vi "CLD 11 Producer consumer events front panel.vi"() -> ()   [LabVIEW 2025]
doc: "CLD 11 exercise"
uses:
  CLD 11 Producer Consumer Data Structure.ctl
  CLD 11 CSV file data structure.ctl
  CLD 11 producer consumer enum.ctl
  CLD 11 CSV file enum.ctl
panel:
  out "Current Time target":dbl
  out "Step 3":bool
  out "Step 2":bool
  out "Step 1":bool
  out "Time Has Elapsed":bool
  out "Elapsed Time":string
  in  "Auto Reset":bool=TRUE
  in  "Reset Button":bool
  in  "Stop VI":bool
  in  "Time Target (s)":dbl
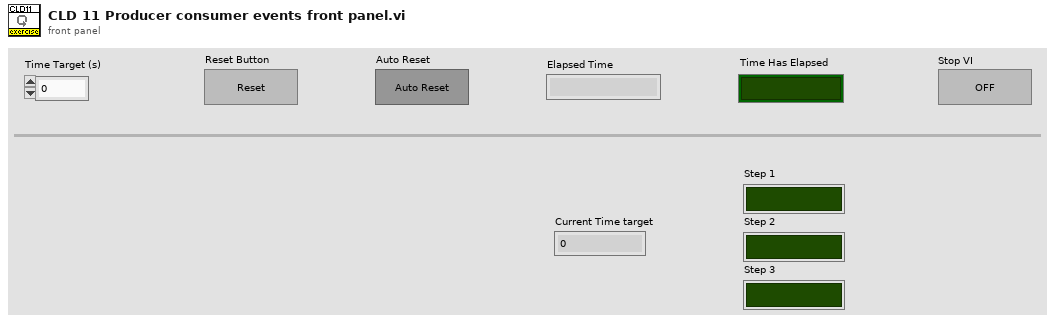
[diagram p1: front panel]
types:
  T1 = typedef "CLD 11 producer consumer enum.ctl" = enum16{"Initialize App", "Read CSV File", "Check Timer", "Run State One", "Run State Two", "Run State Three", "Stop App", "Reset", "Autoreset"}
  T2 = typedef "CLD 11 Producer Consumer Data Structure.ctl" = cluster{"CSV File Data Structure":T3, "Time has Elapsed":bool, "Reset":bool, "Autoreset":bool, "Time Target (s)":dbl, "Current State Number":i32}
  T3 = typedef "CLD 11 CSV file data structure.ctl" = cluster{"Dwell Time":i32, "State 1":bool, "State 2":bool, "State 3":bool}
  T4 = typedef "CLD 11 CSV file enum.ctl" = enum16{"Read CSV", "Write CSV"}
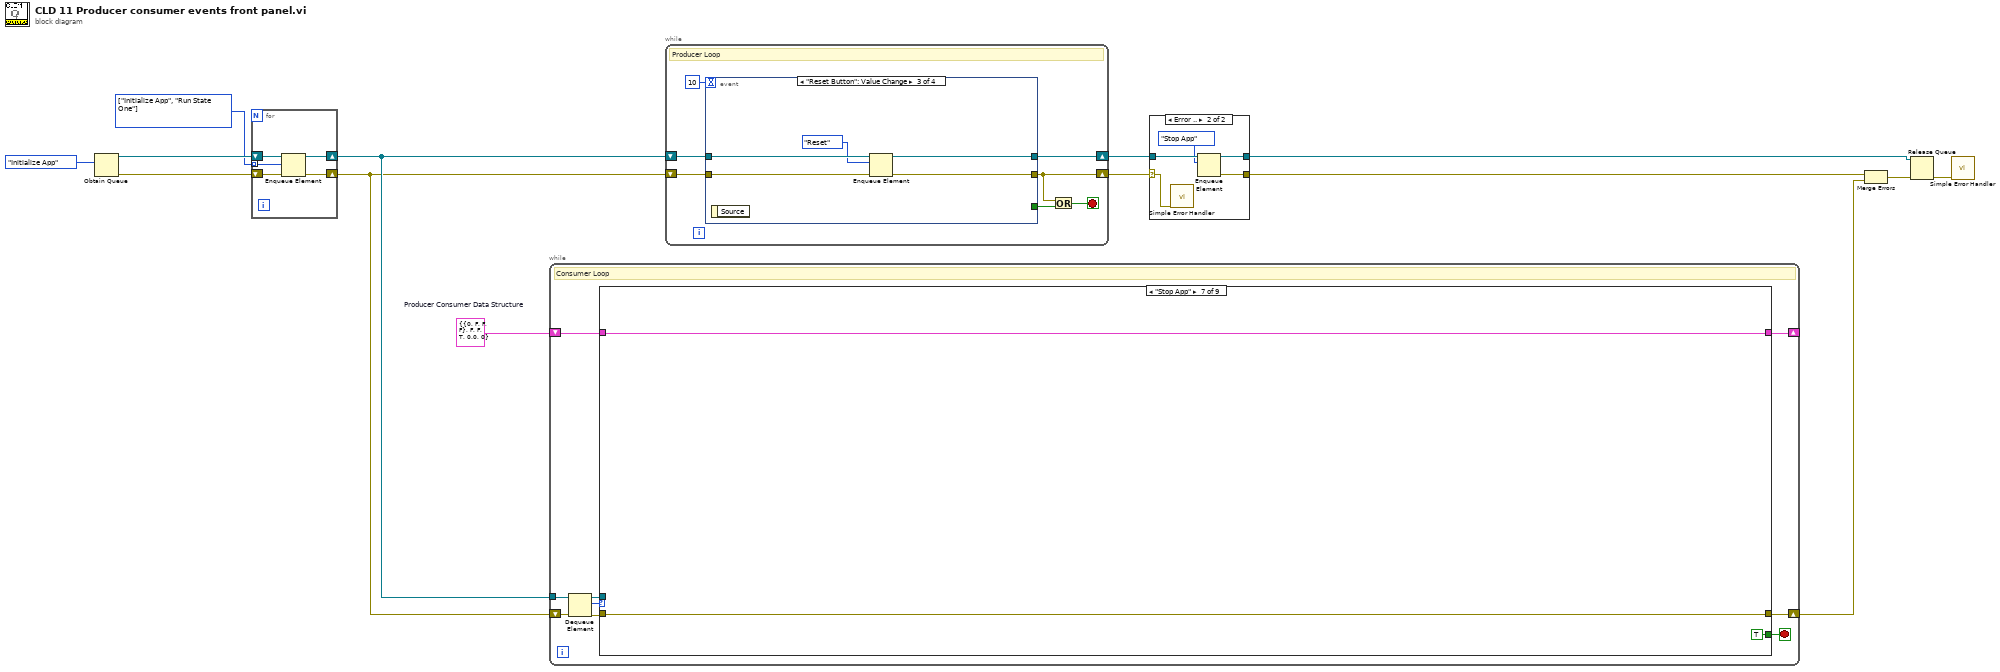
[diagram p0: block diagram]
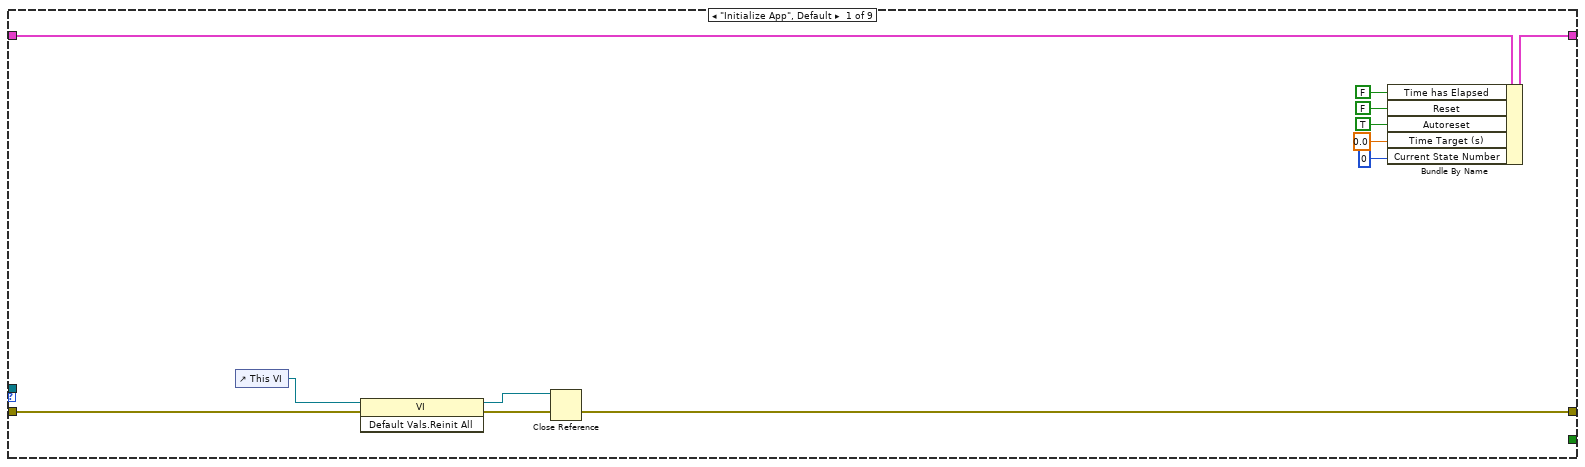
[diagram p3: hidden frame]
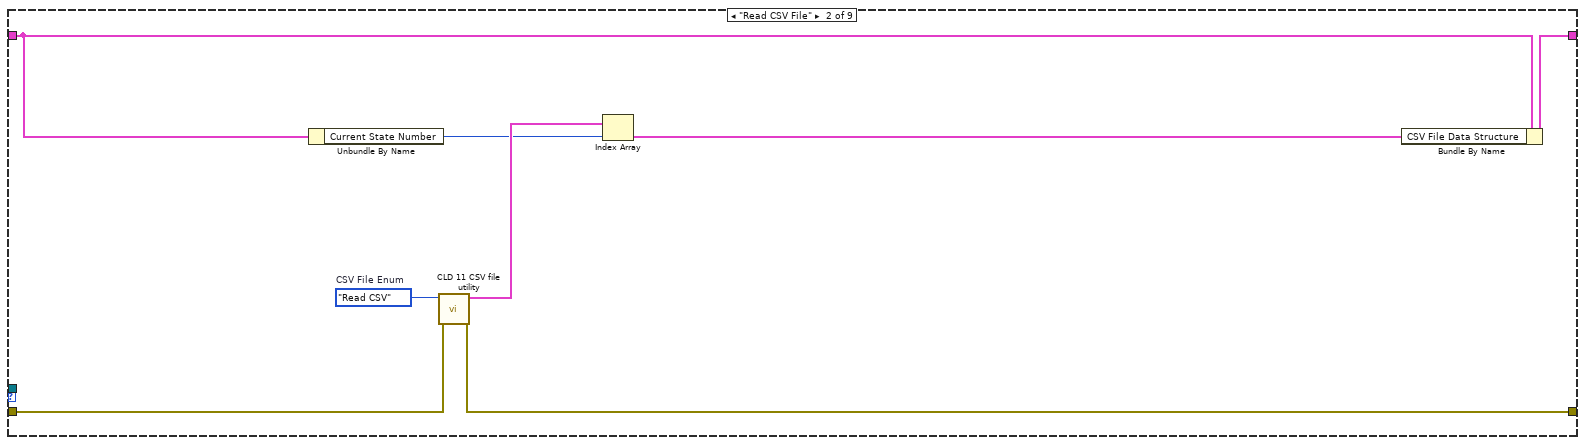
[diagram p4: hidden frame]
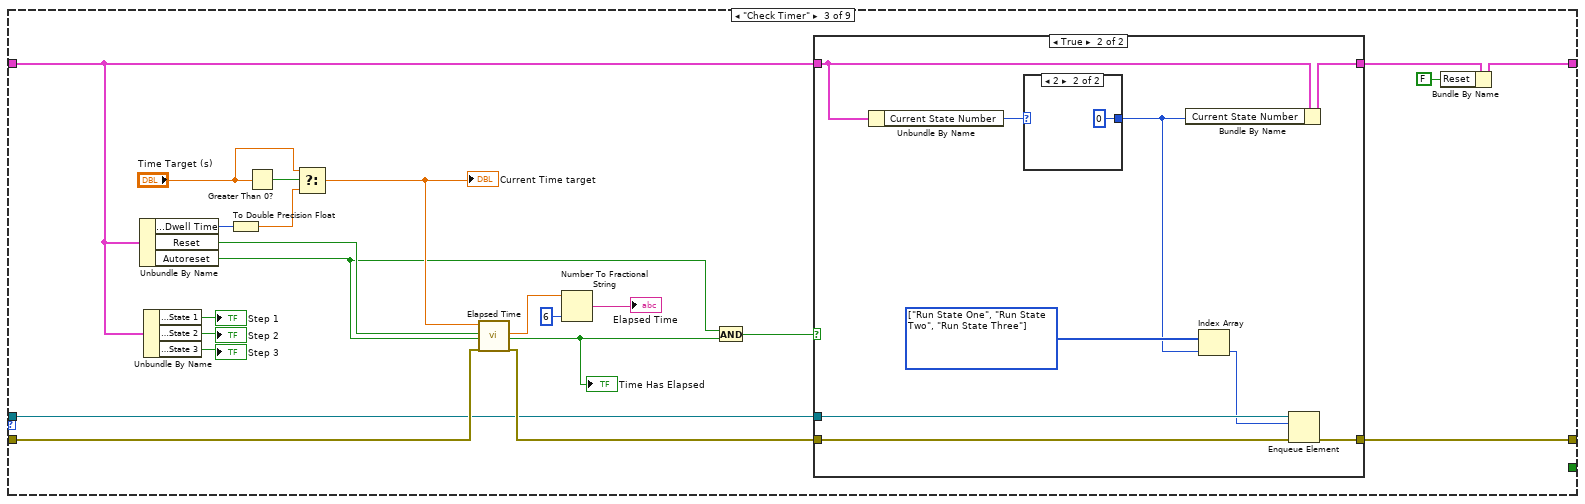
[diagram p5: hidden frame]
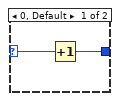
[diagram p7: hidden frame]
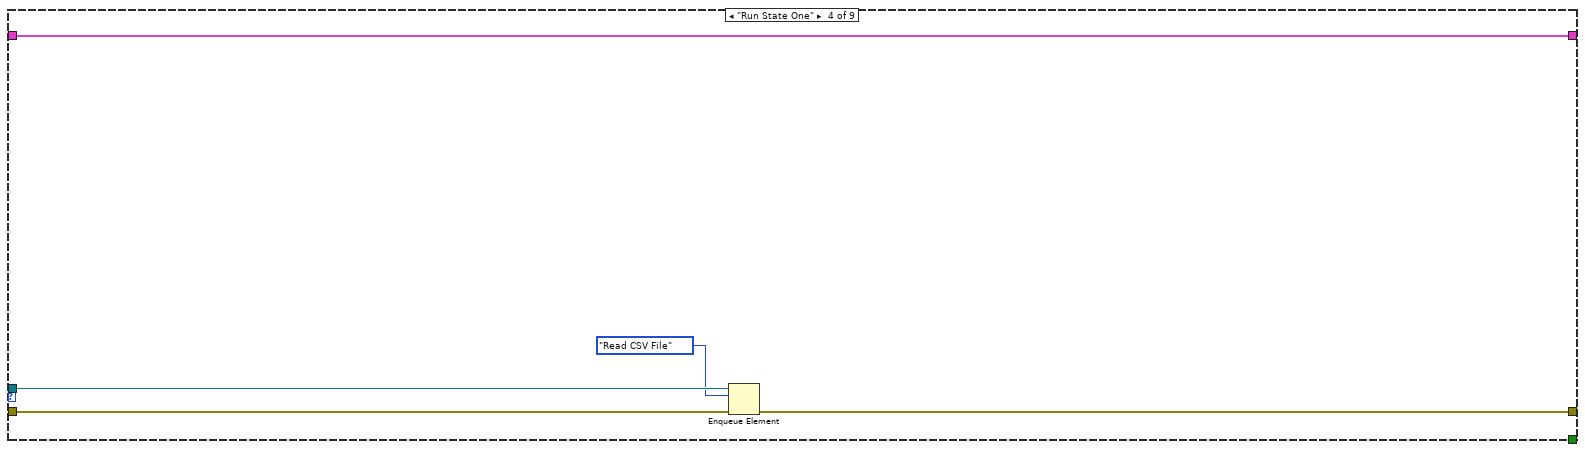
[diagram p8: hidden frame]
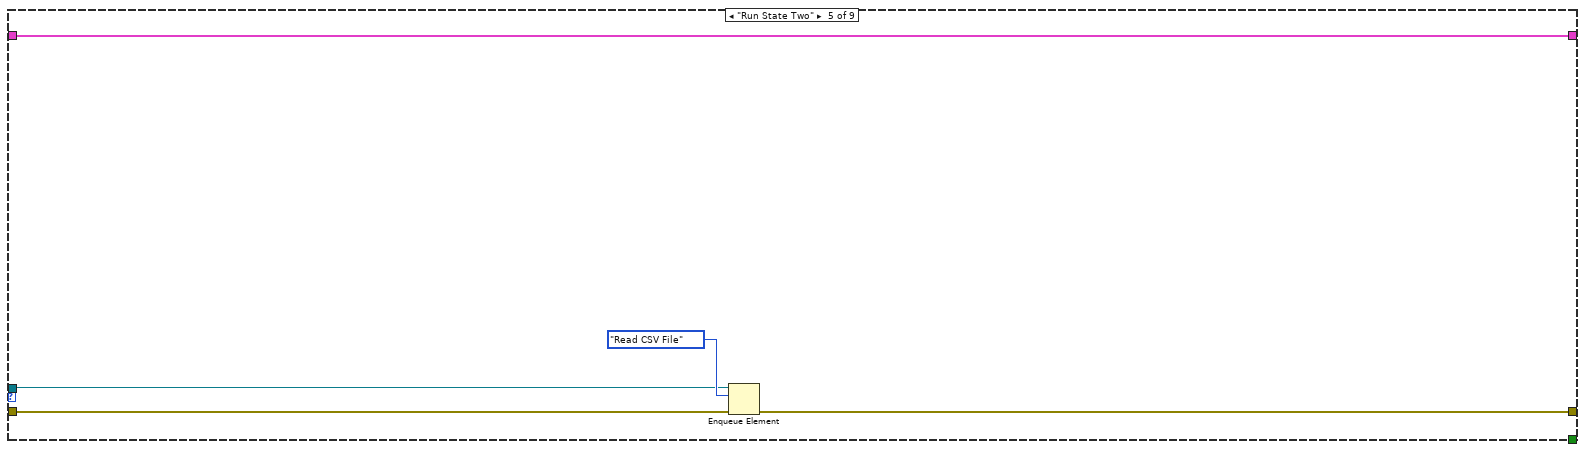
[diagram p9: hidden frame]
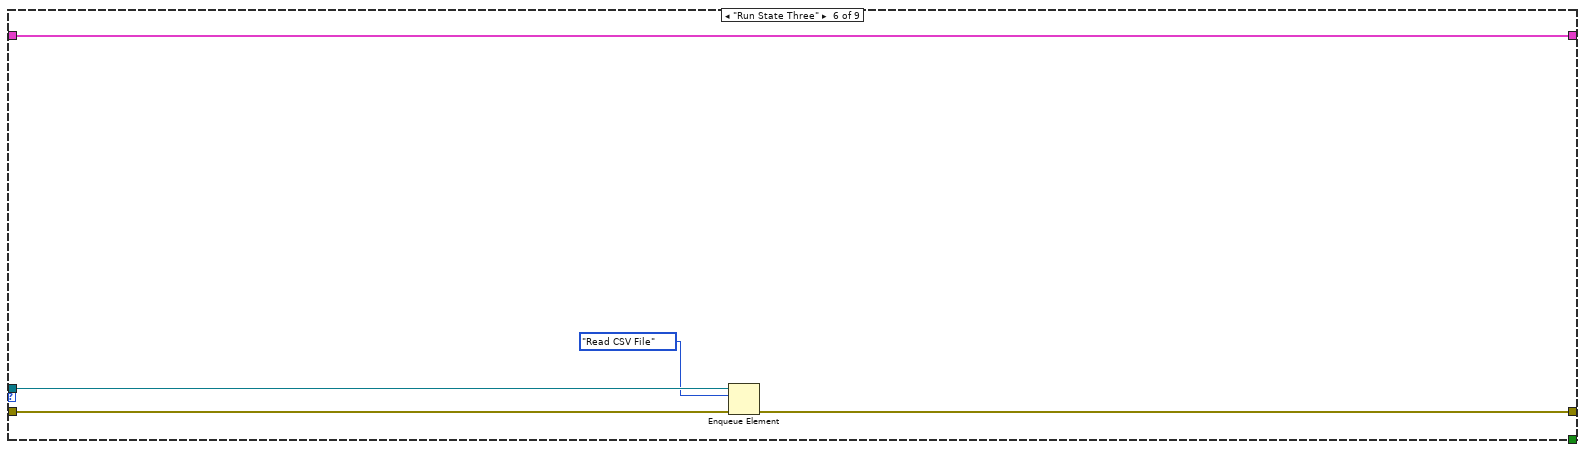
[diagram p10: hidden frame]
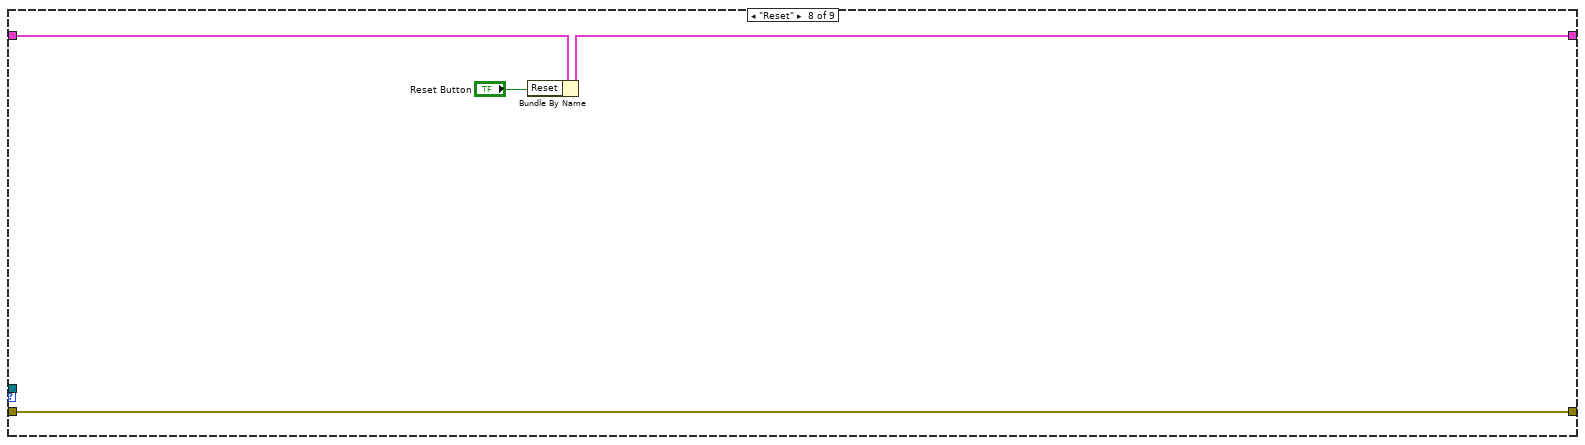
[diagram p11: hidden frame]
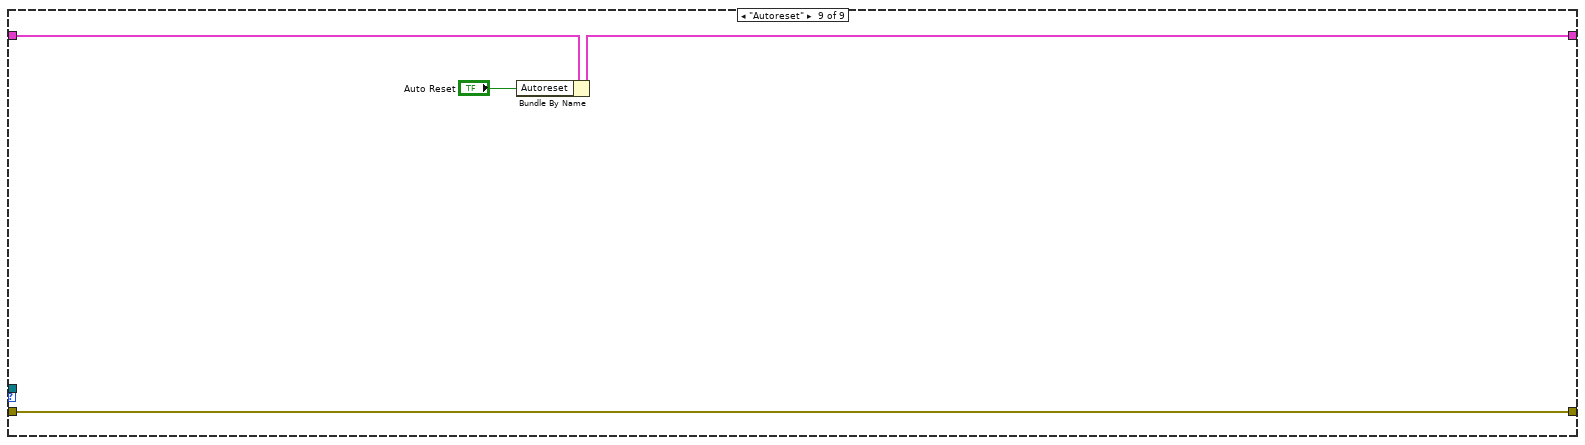
[diagram p12: hidden frame]
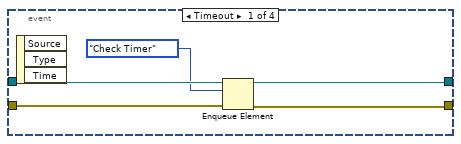
[diagram p13: hidden frame]
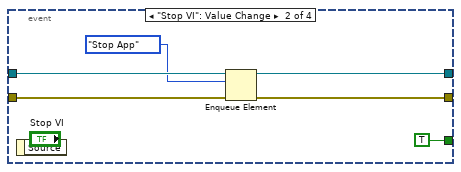
[diagram p14: hidden frame]
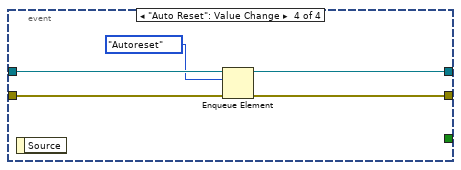
[diagram p15: hidden frame]
diagram:
  w8 = T1[] [enum."Initialize App", enum."Run State One"] items=["Initialize App", "Read CSV File", "Check Timer", "Run State One", "Run State Two", "Run State Three", "Stop App", "Reset", "Autoreset"] ("element")
  w14 = T2 {"CSV File Data Structure"={"Dwell Time"=0, "State 1"=FALSE, "State 2"=FALSE, "State 3"=FALSE}, "Time has Elapsed"=FALSE, "Reset"=FALSE, "Autoreset"=TRUE, "Time Target (s)"=0.0, "Current State Number"=0}  # Producer Consumer Data Structure
  n1 = Obtain Queue(element data type=CLD_11_producer_consumer_enum."Initialize App" ("CLD 11 Timer Enum")) -> (queue out=w11:refnum<queue>, error out=w12:errorcluster)  [unwired: 4 in, 1 out]
  n2 = for {
    shift-right: [w18] -> w9
    shift-left: w12 -> [w19]
    shift-right: [w16] -> w10
    shift-left: w11 -> [w17]
    tunnel: w8 -> [w15] mode=indexing
    n3 = Enqueue Element(queue=w17, element=w15, error in (no error)=w19) -> (queue out=w16:refnum<queue>, error out=w18:errorcluster)  [unwired: 1 in, 1 out]
  }
  n4 = while {
    shift-right: [w26] -> _
    shift-left: w14 -> [w28]
    tunnel: w10 -> [w27]
    shift-right: [w21] -> w7
    shift-left: w9 -> [w23]
    stop <- w24 stop-if-true
    # "Consumer Loop"
    n5 = Dequeue Element(queue=w27, error in (no error)=w23) -> (queue out=w20:refnum<queue>, element=w25:T1, error out=w22:errorcluster)  [unwired: 1 in, 1 out]
    n6 = case shown="\"Stop App\"" w25 {
      tunnel: w28 -> [w40 w44 w55 w90 w95 w97 w103 w107 w111]
      tunnel: [w34 w45 w50 w90 w95 w97 w103 w105 w109] -> w26
      tunnel: [_ _ _ _ _ _ TRUE _ _] -> w24
      tunnel: w22 -> [w39 w48 w71 w89 w94 w100 w101 w106 w110]
      tunnel: [w36 w47 w52 w88 w93 w99 w101 w106 w110] -> w21
      tunnel: w20 -> [_ _ w51 w87 w91 w98 _ _ _]
      frame "Initialize App", Default {
        n7 = control-ref of="This VI"() -> (w37:refnum<vi>)
        n8 = invoke class="VI" method="Default Vals.Reinit All"(reference=w37, error in=w39) -> (reference out=w35:refnum<vi>, error out=w38:errorcluster)  [unwired: 1 in, 1 out]
        n9 = Close Reference(reference=w35, error in (no error)=w38) -> (error out=w36:errorcluster)
        n10 = Bundle By Name(cluster=w40, "Time has Elapsed"=FALSE, "Reset"=FALSE, "Autoreset"=TRUE, "Time Target (s)"=0.0, "Current State Number"=0) -> (w34:T2)
      }
      frame "Read CSV File" {
        w46 = CLD_11_CSV_file_enum."Read CSV"  # CSV File Enum
        n11 = Unbundle By Name(w44) -> ("Current State Number"=w42:i32)
        n12 = call "CLD 11 CSV file utility.vi"("Error In"=w48, "CSV File Enum"=w46) -> ("Error Out"=w47:errorcluster, "[Data Out]"=w43:T3[])  [unwired: 8 in]
        n13 = Index Array(array=w43, index=w42) -> (element=w41:T3)
        n14 = Bundle By Name(cluster=w44, "CSV File Data Structure"=w41) -> (w45:T2)
      }
      frame "Check Timer" {
        n15 = Unbundle By Name(w55) -> ("CSV File Data Structure.Dwell Time"=w61:i32, "Reset"=w64:bool, "Autoreset"=w57:bool)
        n16 = Unbundle By Name(w55) -> ("CSV File Data Structure.State 1"=→"Step 1":bool, "CSV File Data Structure.State 2"=→"Step 2":bool, "CSV File Data Structure.State 3"=→"Step 3":bool)
        n17 = To Double Precision Float(number=w61) -> (double precision float=w60:dbl)
        n18 = Greater Than 0?(x="Time Target (s)") -> (x > 0?=w63:bool)
        n19 = Select(t="Time Target (s)", s=w63, f=w60) -> (s? t:f=w59:dbl)
        "Current Time target" <- w59
        n20 = call "Elapsed Time"("Time Target (s)"=w59, "Reset"=w64, "Auto Reset"=w57, "error in (no error)"=w71) -> ("Elapsed Time (s)"=w66:dbl, "Time has Elapsed"=w58:bool, "error out"=w53:errorcluster)  [unwired: 8 in, 5 out]
        "Time Has Elapsed" <- w58
        n21 = Number To Fractional String(number=w66, precision (6)=i16 6) -> (F-format string=→"Elapsed Time":string)  [unwired: 2 in]
        n22 = And(x=w57, y=w58) -> (x .and. y?=w56:bool)
        n23 = case shown="True" w56 {
          tunnel: w55 -> [w73 w81]
          tunnel: [w73 w82] -> w54
          tunnel: w53 -> [w72 w79]
          tunnel: [w72 w78] -> w52
          tunnel: w51 -> [_ w77]
          frame False {
          }
          frame True {
            w76 = T1[] [enum."Run State One", enum."Run State Two", enum."Run State Three"] items=["Initialize App", "Read CSV File", "Check Timer", "Run State One", "Run State Two", "Run State Three", "Stop App", "Reset", "Autoreset"] ("element")
            n24 = Unbundle By Name(w81) -> ("Current State Number"=w80:i32)
            n25 = case shown="2" w80 {
              selector: w80 -> [w84 _]
              tunnel: [w83 0] -> w75
              frame 0, Default {
                n26 = Increment(x=w84) -> (x+1=w83:i32)
              }
              frame 2 {
              }
            }
            n27 = Bundle By Name(cluster=w81, "Current State Number"=w75) -> (w82:T2)
            n28 = Index Array(array=w76, index=w75) -> (element=w74:T1)
            n29 = Enqueue Element(queue=w77, element=w74, error in (no error)=w79) -> (error out=w78:errorcluster)  [unwired: 1 in, 2 out]
          }
        }
        n30 = Bundle By Name(cluster=w54, "Reset"=FALSE) -> (w50:T2)
      }
      frame "Run State One" {
        n31 = Enqueue Element(queue=w87, element=CLD_11_producer_consumer_enum."Read CSV File", error in (no error)=w89) -> (error out=w88:errorcluster)  [unwired: 1 in, 2 out]
      }
      frame "Run State Two" {
        n32 = Enqueue Element(queue=w91, element=CLD_11_producer_consumer_enum."Read CSV File", error in (no error)=w94) -> (error out=w93:errorcluster)  [unwired: 1 in, 2 out]
      }
      frame "Run State Three" {
        n33 = Enqueue Element(queue=w98, element=CLD_11_producer_consumer_enum."Read CSV File", error in (no error)=w100) -> (error out=w99:errorcluster)  [unwired: 1 in, 2 out]
      }
      frame "Stop App" {
      }
      frame "Reset" {
        n34 = Bundle By Name(cluster=w107, "Reset"="Reset Button") -> (w105:T2)
      }
      frame "Autoreset" {
        n35 = Bundle By Name(cluster=w111, "Autoreset"="Auto Reset") -> (w109:T2)
      }
    }
  }
  n36 = while {
    shift-right: [w114] -> w3
    shift-left: w10 -> [w118]
    shift-right: [w112] -> w5
    shift-left: w9 -> [w117]
    stop <- w113 stop-if-true
    # "Producer Loop"
    n37 = event shown="[2] \"Reset Button\": Value Change" {
      selector: _ -> [_ _ _ _]
      dyn-events: _ -> [_ _ _ _]
      timeout: 10 -> [_ _ _ _]
      tunnel: w118 -> [w122 w129 w134 w138]
      tunnel: w117 -> [w123 w128 w133 w139]
      tunnel: [_ TRUE _ _] -> w116
      tunnel: [w119 w124 w130 w136] -> w112
      tunnel: [w120 w125 w131 w135] -> w114
      event Timeout {
        n38 = event-data() -> ()  [unwired: 1 in, 3 out]
        n39 = Enqueue Element(queue=w122, element=CLD_11_producer_consumer_enum."Check Timer", error in (no error)=w123) -> (queue out=w120:refnum<queue>, error out=w119:errorcluster)  [unwired: 1 in, 1 out]
      }
      event "Stop VI": Value Change {
        n40 = event-data() -> ()  [unwired: 1 in, 1 out]
        n41 = Enqueue Element(queue=w129, element=CLD_11_producer_consumer_enum."Stop App" ("CLD 11 Timer Enum"), error in (no error)=w128) -> (queue out=w125:refnum<queue>, error out=w124:errorcluster)  [unwired: 1 in, 1 out]
      }
      event "Reset Button": Value Change {
        n42 = event-data() -> ()  [unwired: 1 in, 1 out]
        n43 = Enqueue Element(queue=w134, element=CLD_11_producer_consumer_enum."Reset", error in (no error)=w133) -> (queue out=w131:refnum<queue>, error out=w130:errorcluster)  [unwired: 1 in, 1 out]
      }
      event "Auto Reset": Value Change {
        n44 = event-data() -> ()  [unwired: 1 in, 1 out]
        n45 = Enqueue Element(queue=w138, element=CLD_11_producer_consumer_enum."Autoreset", error in (no error)=w139) -> (queue out=w135:refnum<queue>, error out=w136:errorcluster)  [unwired: 1 in, 1 out]
      }
    }
    n46 = Or(x=w112, y=w116) -> (x .or. y?=w113:bool)
  }
  n47 = case shown="Error .." w5 {
    selector: w5 -> [w141 w142]
    tunnel: [w141 w146] -> w4
    tunnel: w3 -> [w140 w145]
    tunnel: [w140 w143] -> w1
    frame No Error {
    }
    frame Error {
      n48 = call <vilib>:"Simple Error Handler.vi"("error in (no error)"=w142) -> ()  [unwired: 4 in, 5 out]
      n49 = Enqueue Element(queue=w145, element=CLD_11_producer_consumer_enum."Stop App") -> (queue out=w143:refnum<queue>, error out=w146:errorcluster)  [unwired: 2 in, 1 out]
    }
  }
  n50 = Merge Errors(w4, w7) -> (w6:errorcluster)
  n51 = Release Queue(queue=w1, error in (no error)=w6) -> (error out=w2:errorcluster)  [unwired: 1 in, 2 out]
  n52 = call <vilib>:"Simple Error Handler.vi"("error in (no error)"=w2) -> ()  [unwired: 4 in, 5 out]
